vi "MSEncoder Case-42-UpdAO.vi"(8 "error in (no error)":errorcluster, 9 "ParamValIn":variant, 11 "MSEncoder in":refnum<class "MSEncoder.lvclass">) -> (0 "error out":errorcluster, 3 "MSEncoder out":refnum<class "MSEncoder.lvclass">)   [LabVIEW 2018, in "MSEncoder.lvclass"]
uses:
  MSEncoder.lvclass
  Ctl/MSEditorParam updAO.ctl
  MSEncoder.lvclass/MSEncoder.ctl
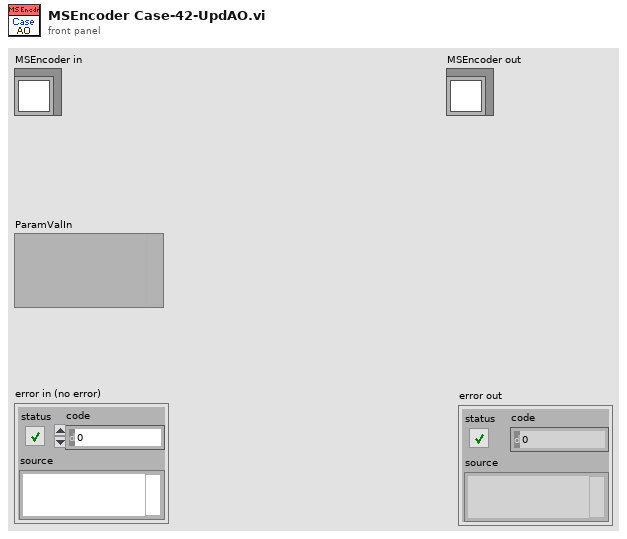
[diagram p1: front panel]
types:
  T1 = typedef "MSEditorParam updAO.ctl" = cluster{"func":u32[], "val":ext[]}
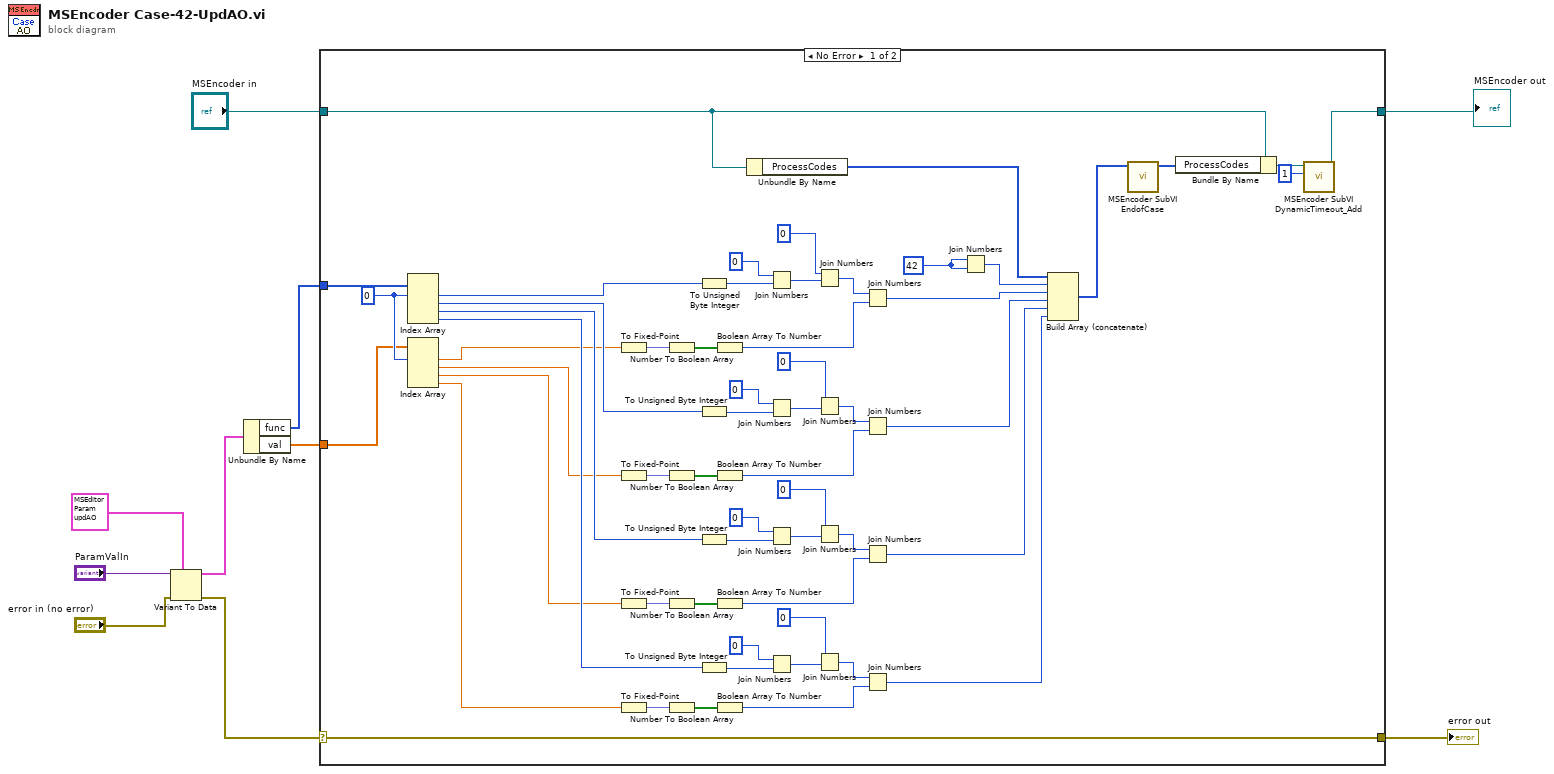
[diagram p0: block diagram]
diagram:
  n1 = Variant To Data(error in="error in (no error)", type=T1 {"func"=[0, 0, 0, 0], "val"=[0.0, 0.0, 0.0, 0.0]} ("ParamValueType"), Variant="ParamValIn") -> (data=w2:T1, error out=w3:errorcluster)
  n2 = Unbundle By Name(w2) -> ("func"=w9:u32[], "val"=w8:ext[])
  n3 = case shown="No Error" w3 {
    selector: w3 -> [w66 w69]
    tunnel: "MSEncoder in" -> [w65 w68]
    tunnel: [w66 w69] -> w10
    tunnel: [w12 w68] -> w7
    tunnel: w9 -> [w14 _]
    tunnel: w8 -> [w15 _]
    frame No Error {
      w20 = 0 ("index")
      w63 = u32 42
      n4 = Index Array(array=w14, index #1=w20) -> (element #1=w24:u32, element #2=w23:u32, element #3=w22:u32, element #4=w21:u32)  [unwired: 3 in]
      n5 = Index Array(array=w15, index #1=w20) -> (element #1=w19:ext, element #2=w18:ext, element #3=w17:ext, element #4=w16:ext)  [unwired: 3 in]
      n6 = To Fixed-Point(number=w19) -> (fixed-point=w58:fxp<+/-,32,5>)  [unwired: 1 in]
      n7 = To Fixed-Point(number=w18) -> (fixed-point=w47:fxp<+/-,32,5>)  [unwired: 1 in]
      n8 = To Fixed-Point(number=w17) -> (fixed-point=w31:fxp<+/-,32,5>)  [unwired: 1 in]
      n9 = To Fixed-Point(number=w16) -> (fixed-point=w42:fxp<+/-,32,5>)  [unwired: 1 in]
      n10 = Number To Boolean Array(number=w58) -> (Boolean array=w59:bool[])
      n11 = Number To Boolean Array(number=w47) -> (Boolean array=w46:bool[])
      n12 = Number To Boolean Array(number=w31) -> (Boolean array=w30:bool[])
      n13 = Number To Boolean Array(number=w42) -> (Boolean array=w43:bool[])
      n14 = To Unsigned Byte Integer(number=w24) -> (unsigned 8bit integer=w25:u8)
      n15 = To Unsigned Byte Integer(number=w23) -> (unsigned 8bit integer=w45:u8)
      n16 = To Unsigned Byte Integer(number=w22) -> (unsigned 8bit integer=w29:u8)
      n17 = To Unsigned Byte Integer(number=w21) -> (unsigned 8bit integer=w44:u8)
      n18 = Boolean Array To Number(Boolean array=w59) -> (number=w53:u32)
      n19 = Boolean Array To Number(Boolean array=w46) -> (number=w52:u32)
      n20 = Boolean Array To Number(Boolean array=w30) -> (number=w36:u32)
      n21 = Boolean Array To Number(Boolean array=w43) -> (number=w37:u32)
      n22 = Unbundle By Name(w65) -> ("ProcessCodes"=w67:u64[])
      n23 = Join Numbers(hi=u8 0, lo=w25) -> ((hi.lo)=w57:u16)
      n24 = Join Numbers(hi=u8 0, lo=w45) -> ((hi.lo)=w48:u16)
      n25 = Join Numbers(hi=u8 0, lo=w29) -> ((hi.lo)=w32:u16)
      n26 = Join Numbers(hi=u8 0, lo=w44) -> ((hi.lo)=w41:u16)
      n27 = Join Numbers(hi=u16 0, lo=w57) -> ((hi.lo)=w54:u32)
      n28 = Join Numbers(hi=u16 0, lo=w48) -> ((hi.lo)=w51:u32)
      n29 = Join Numbers(hi=u16 0, lo=w32) -> ((hi.lo)=w35:u32)
      n30 = Join Numbers(hi=u16 0, lo=w41) -> ((hi.lo)=w38:u32)
      n31 = Join Numbers(hi=w54, lo=w53) -> ((hi.lo)=w61:u64)
      n32 = Join Numbers(hi=w51, lo=w52) -> ((hi.lo)=w28:u64)
      n33 = Join Numbers(hi=w35, lo=w36) -> ((hi.lo)=w27:u64)
      n34 = Join Numbers(hi=w38, lo=w37) -> ((hi.lo)=w26:u64)
      n35 = Join Numbers(hi=w63, lo=w63) -> ((hi.lo)=w62:u64)
      n36 = Build Array (concatenate)(w67, w62, w61, w28, w27, w26) -> (w60:u64[])
      n37 = call "MSEncoder SubVI EndofCase.vi"("Case codes"=w60) -> ("Case codes with end"=w64:u64[])  [unwired: 9 in, 1 out]
      n38 = Bundle By Name(cluster=w65, "ProcessCodes"=w64) -> (w13:refnum<class "MSEncoder.lvclass">)
      n39 = call "MSEncoder SubVI DynamicTimeout_Add.vi"("Timeout_ms"=1, "MSEncoder"=w13) -> ("MSEncoder"=w12:refnum<class "MSEncoder.lvclass">)  [unwired: 8 in, 1 out]
    }
    frame Error {
    }
  }
  "error out" <- w10
  "MSEncoder out" <- w7
